vi "unescape json string 2.vi"(9 "quotes removed?":bool, 11 "base string":string) -> (3 "String out":string)   [LabVIEW 2013]
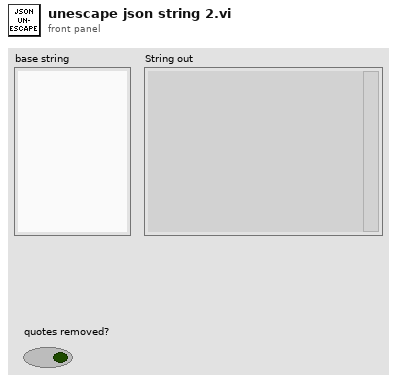
[diagram p1: front panel]
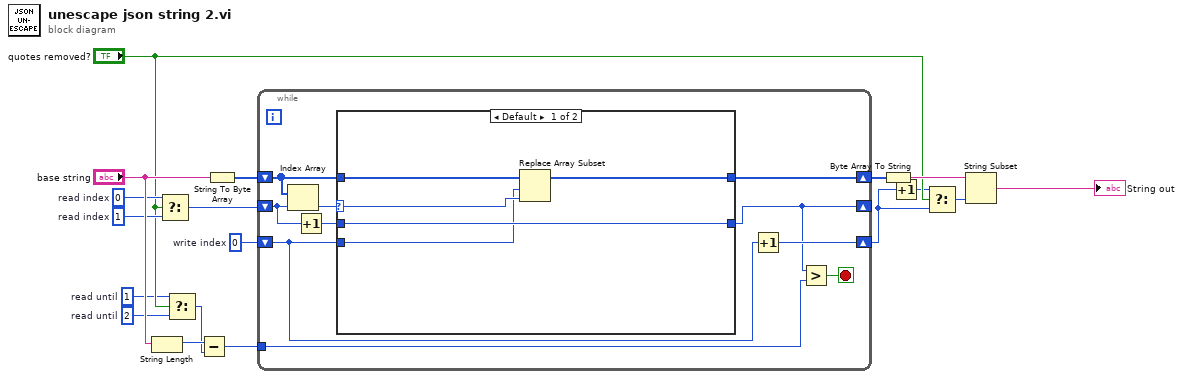
[diagram p0: block diagram]
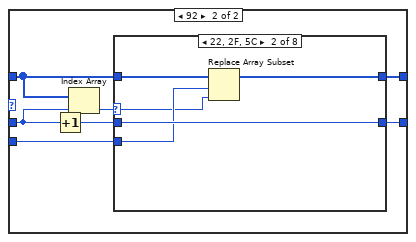
[diagram p2: hidden frame]
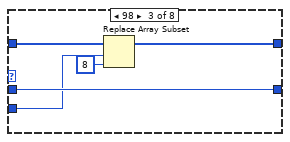
[diagram p4: hidden frame]
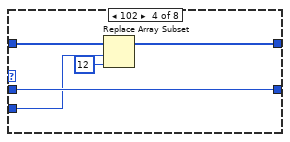
[diagram p5: hidden frame]
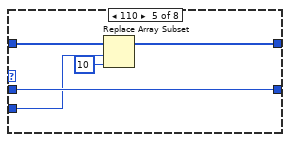
[diagram p6: hidden frame]
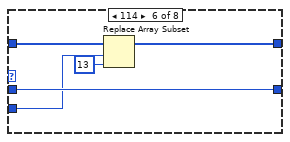
[diagram p7: hidden frame]
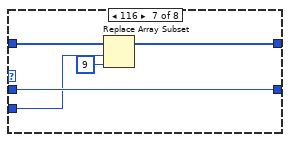
[diagram p8: hidden frame]
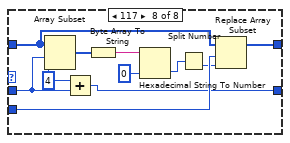
[diagram p9: hidden frame]
diagram:
  w4 = 1  # read until
  w3 = 2  # read until
  w12 = 0  # read index
  w11 = 1  # read index
  w14 = 0  # write index
  n1 = String Length(string="base string") -> (length=w6:i32)
  n2 = Select(t=w12, s="quotes removed?", f=w11) -> (s? t:f=w10:i32)
  n3 = Select(t=w4, s="quotes removed?", f=w3) -> (s? t:f=w5:i32)
  n4 = Subtract(x=w6, y=w5) -> (x-y=w2:i32)
  n5 = String To Byte Array(string="base string") -> (unsigned byte array=w16:u8[])
  n6 = while {
    shift-right: [w26] -> w13
    shift-left: w16 -> [w27]
    shift-right: [w19] -> _
    shift-left: w10 -> [w23]
    shift-right: [w20] -> w8
    shift-left: w14 -> [w24]
    tunnel: w2 -> [w21]
    stop <- w22 stop-if-true
    n7 = Index Array(array=w27, index=w23) -> (element=w28:u8)
    n8 = Increment(x=w23) -> (x+1=w25:i32)
    n9 = case shown="Default" w28 {
      selector: w28 -> [w30 _]
      tunnel: w27 -> [w33 w39]
      tunnel: [w31 w38] -> w26
      tunnel: w25 -> [w32 w36]
      tunnel: w24 -> [w29 w37]
      tunnel: [w32 w35] -> w19
      frame Default {
        n10 = Replace Array Subset(array=w33, new element=w30, index=w29) -> (w31:u8[])
      }
      frame 92 {
        n11 = Increment(x=w36) -> (x+1=w34:i32)
        n12 = Index Array(array=w39, index=w36) -> (element=w40:u8)
        n13 = case shown="22, 2F, 5C" w40 {
          selector: w40 -> [_ w43 _ _ _ _ _ _]
          tunnel: w39 -> [w42 w47 w52 w57 w62 w67 w72 w80]
          tunnel: [w42 w46 w51 w56 w61 w66 w71 w81] -> w38
          tunnel: w37 -> [_ w44 w49 w54 w59 w64 w69 w79]
          tunnel: w34 -> [w41 w45 w50 w55 w60 w65 w70 w82]
          tunnel: [w41 w45 w50 w55 w60 w65 w70 w78] -> w35
          frame Default {
            # "error"
          }
          frame 34, 47, 92 {
            n14 = Replace Array Subset(array=w47, new element=w43, index=w44) -> (w46:u8[])
          }
          frame 98 {
            n15 = Replace Array Subset(array=w52, new element=u8 8 ("new element/subarray"), index=w49) -> (w51:u8[])
          }
          frame 102 {
            n16 = Replace Array Subset(array=w57, new element=u8 12 ("new element/subarray"), index=w54) -> (w56:u8[])
          }
          frame 110 {
            n17 = Replace Array Subset(array=w62, new element=u8 10 ("new element/subarray"), index=w59) -> (w61:u8[])
          }
          frame 114 {
            n18 = Replace Array Subset(array=w67, new element=u8 13 ("new element/subarray"), index=w64) -> (w66:u8[])
          }
          frame 116 {
            n19 = Replace Array Subset(array=w72, new element=u8 9 ("new element/subarray"), index=w69) -> (w71:u8[])
          }
          frame 117 {
            w83 = 4 ("length")
            n20 = Array Subset(array=w80, index=w82, length=w83) -> (w77:u8[])
            n21 = Add(x=w83, y=w82) -> (x+y=w78:i32)
            n22 = Byte Array To String(unsigned byte array=w77) -> (string=w76:string)
            n23 = Hexadecimal String To Number(string=w76, default (0uL)=u16 0 ("default (0 U32)")) -> (number=w74:u16)  [unwired: 1 in, 1 out]
            n24 = Split Number(x=w74) -> (lo(x)=w73:u8)  [unwired: 1 out]
            n25 = Replace Array Subset(array=w80, new element=w73, index=w79) -> (w81:u8[])
          }
        }
      }
    }
    n26 = Increment(x=w24) -> (x+1=w20:i32)
    n27 = Greater?(x=w19, y=w21) -> (0:w22:bool)
  }
  n28 = Byte Array To String(unsigned byte array=w13) -> (string=w15:string)
  n29 = Increment(x=w8) -> (x+1=w1:i32)
  n30 = Select(t=w1, s="quotes removed?", f=w8) -> (s? t:f=w9:i32)
  n31 = String Subset(string=w15, length (rest)=w9) -> (substring=→"String out":string)  [unwired: 1 in]
